vi "change_stored_position.vi"(5 "Row":i32, 6 "String":string, 7 "Column":i32, 8 "error in (no error)":errorcluster, 9 "specific class reference":refnum<class "StageDL090409Scaffold.lvclass">, 11 "StageDL090409Scaffold in":refnum<class "StageDL090409Scaffold.lvclass">) -> (0 "error out":errorcluster, 1 "specific class reference out":refnum<class "StageDL090409Scaffold.lvclass">, 3 "StageDL090409Scaffold out":refnum<class "StageDL090409Scaffold.lvclass">)   [LabVIEW 2010, in "StageDL090409Scaffold.lvclass"]
uses:
  StageDL090409Scaffold.lvclass
  StageDL090409Scaffold.lvclass/StageDL090409Scaffold.ctl
  common/classes/SpaceVector/SpaceVector/SpaceVector.lvclass
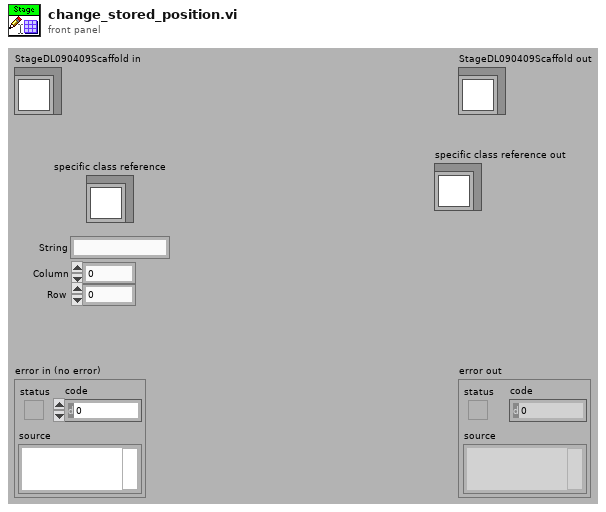
[diagram p1: front panel]
types:
  T1 = typedef "StageDL090409Scaffold.lvclass/stored_data_cluster.ctl" = cluster{"stored position":refnum<class "SpaceVector.lvclass">, "description":string, "position image":refnum<class "Image.lvclass">}
  T2 = typedef "space_vector_array.ctl" = dbl[unit][]
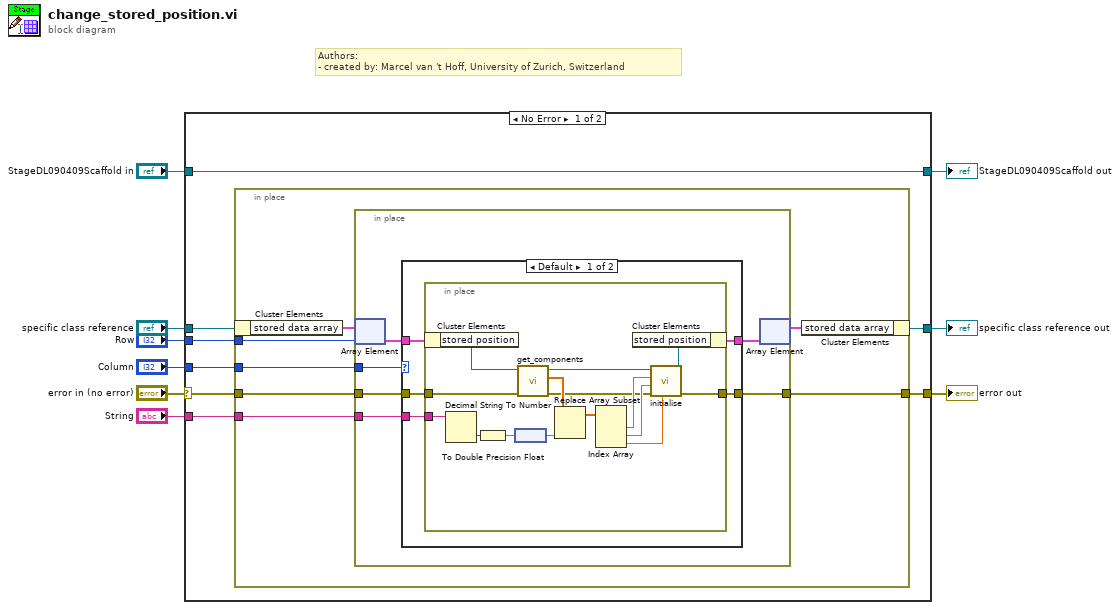
[diagram p0: block diagram]
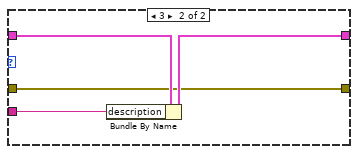
[diagram p2: hidden frame]
diagram:
  # "Authors: \n- created by: Marcel van 't Hoff, University of Zurich, Switzerland"
  n1 = case shown="No Error" "error in (no error)" {
    selector: "error in (no error)" -> [w12 w57]
    tunnel: [w10 w57] -> w8
    tunnel: [w17 w56] -> w6
    tunnel: "StageDL090409Scaffold in" -> [w17 w56]
    tunnel: "specific class reference" -> [w16 w55]
    tunnel: "Row" -> [w15 _]
    tunnel: "Column" -> [w14 _]
    tunnel: "String" -> [w13 _]
    tunnel: [w11 w55] -> w1
    frame No Error {
      n2 = in-place {
        in-place-border: w13 -> [w21]
        in-place-border: w15 -> [w23]
        in-place-border: w14 -> [w20]
        in-place-border: w12 -> [w19]
        in-place-border: [w18] -> w10
        n3 = in-place-cluster #1(w16) -> ("stored data array"=w24:T1[])
        n4 = in-place {
          in-place-border: w21 -> [w29]
          in-place-border: w20 -> [w30]
          in-place-border: w19 -> [w26]
          in-place-border: [w25] -> w18
          n5 = in-place-array #2(w24, w23) -> (w28:T1)
          n6 = case shown="Default" w30 {
            tunnel: w29 -> [w34 w54]
            tunnel: w28 -> [w35 w53]
            tunnel: [w33 w52] -> w27
            tunnel: w26 -> [w32 w51]
            tunnel: [w31 w51] -> w25
            frame Default {
              n7 = in-place {
                in-place-border: w34 -> [w48]
                in-place-border: w32 -> [w37]
                in-place-border: [w36] -> w31
                n8 = in-place-cluster #3(w35) -> ("stored position"=w45:refnum<class "SpaceVector.lvclass">)
                n9 = Decimal String To Number(string=w48) -> (number=w50:i32)  [unwired: 2 in, 1 out]
                n10 = To Double Precision Float(number=w50) -> (double precision float=w49:dbl)
                n11 = node(w49) -> (w43:dbl[unit])
                n12 = call "get_components.vi"("error in (no error)"=w37, "SpaceVector in"=w45) -> ("error out"=w38:errorcluster, "x/y/z"=w46:T2, "SpaceVector out"=w44:refnum<class "SpaceVector.lvclass">)  [unwired: 4 in, 3 out]
                n13 = Replace Array Subset(array=w46, new element=w43) -> (w47:T2)  [unwired: 1 in]
                n14 = Index Array(array=w47) -> (element #1=w42:dbl[unit], element #2=w41:dbl[unit], element #3=w40:dbl[unit])  [unwired: 3 in]
                n15 = call "initialise.vi"("z"=w40, "error in (no error)"=w38, "y"=w41, "x"=w42, "SpaceVector in"=w44) -> ("error out"=w36:errorcluster, "SpaceVector out"=w39:refnum<class "SpaceVector.lvclass">)  [unwired: 5 in]
                n16 = in-place-cluster #3("stored position"=w39) -> (w33:T1)
              }
            }
            frame 3 {
              n17 = Bundle By Name(cluster=w53, "description"=w54) -> (w52:T1)
            }
          }
          n18 = in-place-array #2(w27) -> (w22:T1[])  [unwired: 1 out]
        }
        n19 = in-place-cluster #1("stored data array"=w22) -> (w11:refnum<class "StageDL090409Scaffold.lvclass">)
      }
    }
    frame Error {
    }
  }
  "error out" <- w8
  "StageDL090409Scaffold out" <- w6
  "specific class reference out" <- w1
